vi "Test_Switch.vi"(2 "TestModel":T1, 3 "error in (no error)":errorcluster, 4 "Contactor":refnum<k21>, 5 "Break":refnum<k21>) -> (0 "error out":errorcluster, 1 "Break":bool[](array[boolean]))   [LabVIEW 2015]
uses:
  CustomControl/Model.ctl
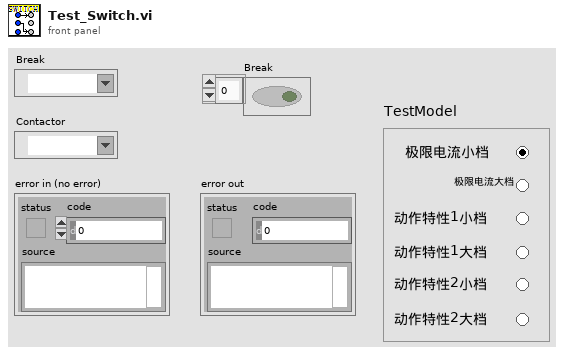
[diagram p1: front panel]
types:
  T1 = typedef "Model.ctl" = enum32{"lowLimit", "upLimit", "lowAction1", "upAction1", "lowAction2", "upAction2"}
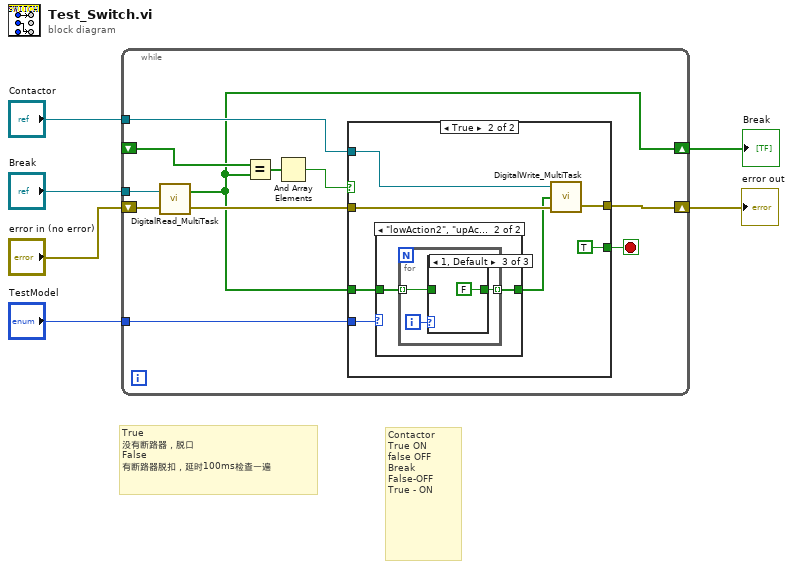
[diagram p0: block diagram]
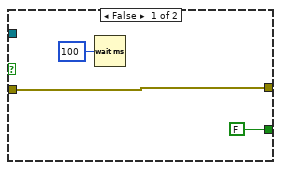
[diagram p2: hidden frame]
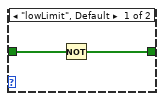
[diagram p3: hidden frame]
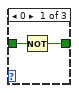
[diagram p4: hidden frame]
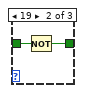
[diagram p5: hidden frame]
diagram:
  # "Contactor\nTrue ON\nfalse OFF\nBreak\nFalse-OFF\nTrue - ON"
  # "True\n没有断路器，脱口\nFalse\n有断路器脱扣，延时100ms检查一遍"
  n1 = while {
    shift-right: [w8] -> w3
    shift-left: _ -> [w15]
    tunnel: "Contactor" -> [w13]
    shift-right: [w12] -> w4
    shift-left: "error in (no error)" -> [w11]
    tunnel: "Break" -> [w10]
    tunnel: "TestModel" -> [w7]
    stop <- w17 stop-if-true
    n2 = call "DigitalRead_MultiTask.vi"("error in"=w11, "mutiTask"=w10) -> ("error out"=w9:errorcluster, "read"=w8:bool[])
    n3 = Equal?(x=w15, y=w8) -> (x = y?=w16:bool[])
    n4 = And Array Elements(Boolean array=w16) -> (logical AND=w14:bool)
    n5 = case shown="True" w14 {
      tunnel: [FALSE TRUE] -> w17
      tunnel: w9 -> [w18 w24]
      tunnel: w13 -> [_ w25]
      tunnel: [w18 w26] -> w12
      tunnel: w8 -> [_ w23]
      tunnel: w7 -> [_ w21]
      frame False {
        n6 = Wait (ms)(milliseconds to wait=u32 100) -> ()  [unwired: 1 out]
      }
      frame True {
        n7 = case shown="\"lowAction2\", \"upAction2\"" w21 {
          tunnel: w23 -> [w29 w31]
          tunnel: [w28 w30] -> w22
          frame "lowLimit", Default {
            n8 = Not(x=w29) -> (.not. x?=w28:bool[])
          }
          frame "lowAction2", "upAction2" {
            n9 = for {
              tunnel: w31 -> [w33] mode=indexing
              tunnel: [w32] -> w30 mode=indexing
              i -> [w34]
              n10 = case shown="1, Default" w34 {
                tunnel: w33 -> [w36 w38 _]
                tunnel: [w35 w37 FALSE ("Boolean")] -> w32
                frame 0 {
                  n11 = Not(x=w36) -> (.not. x?=w35:bool)
                }
                frame 19 {
                  n12 = Not(x=w38) -> (.not. x?=w37:bool)
                }
                frame 1, Default {
                }
              }
            }
          }
        }
        n13 = call "DigitalWrite_MultiTask.vi"("error in"=w24, "input"=w22, "mutiTask"=w25) -> ("error out"=w26:errorcluster)  [unwired: 1 in]
      }
    }
  }
  "error out" <- w4
  "Break" <- w3
